vi "CLD 2  Elapsed Time Express with pause Front Panel.vi"() -> ()   [LabVIEW 2009]
doc: "CLD-Zusatzaufgabe 2"
panel:
  out "Verstrichene Zeit (s)":dbl
  out "Zeit ist verstrichen":bool
  in  "Autom. zurücksetzen":bool
  in  "Pause-Schaltfläche":bool
  in  "Zurücksetzen-Schaltfläche":bool
  in  "VI anhalten":bool
  out "Fehler (Ausgang)":errorcluster
  in  "Fehler (Eingang, kein Fehler)":errorcluster
  in  "Zielzeit (s)":dbl
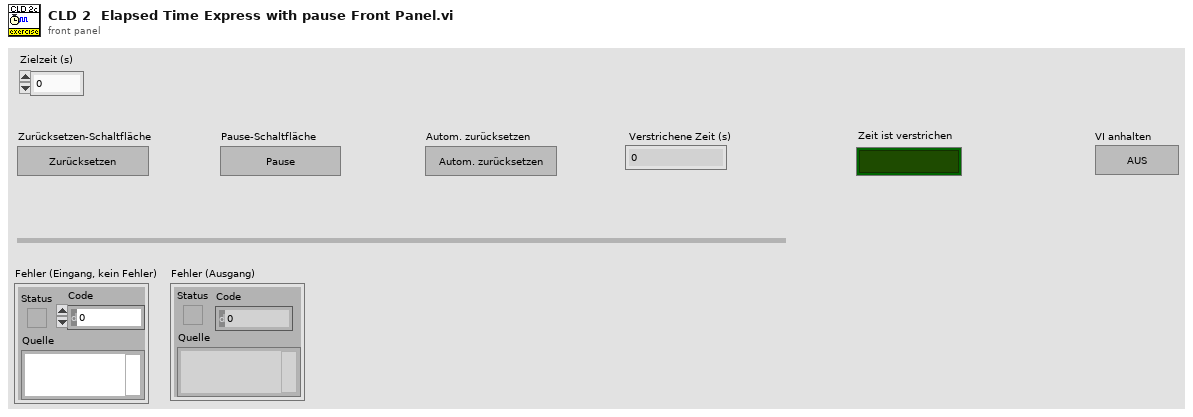
[diagram p1: front panel]
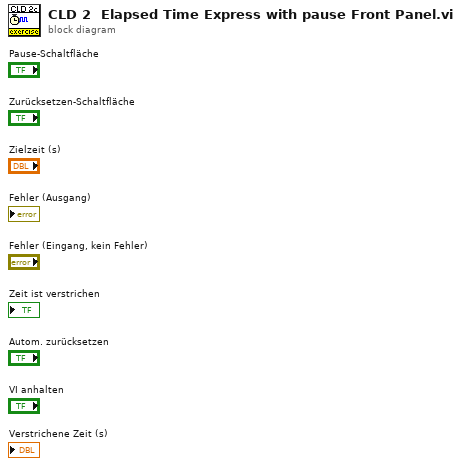
[diagram p0: block diagram]
diagram:
